vi "Lire_n_splits.vi"(8 "error in (no error)":errorcluster caption="entrée d'erreur (pas d'erreur)", 11 "Splitter en entrée":refnum<class "Splitter.lvclass">) -> (0 "error out":errorcluster caption="sortie d'erreur", 2 "n_splits":u8, 3 "Splitter en sortie":refnum<class "Splitter.lvclass">)   [LabVIEW 2020, in "Splitter.lvclass"]
uses:
  Splitter.lvclass
  Splitter.lvclass/Splitter.ctl
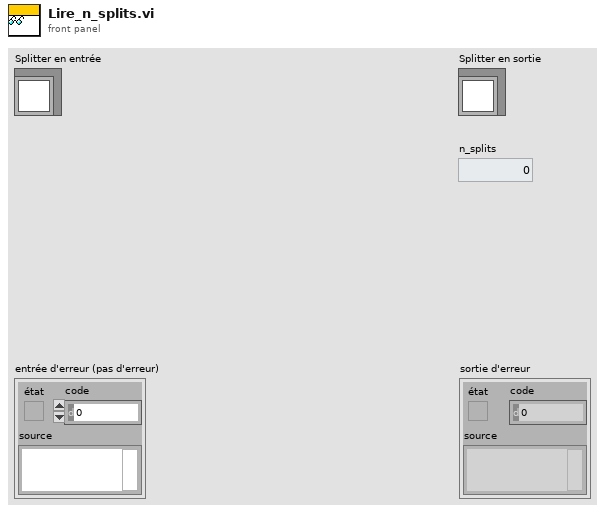
[diagram p1: front panel]
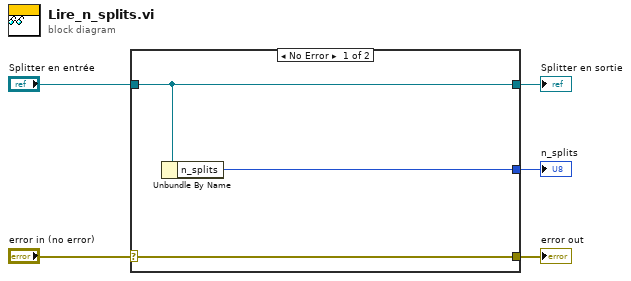
[diagram p0: block diagram]
diagram:
  n1 = case shown="No Error" "error in (no error)" {
    selector: "error in (no error)" -> [w8 w9]
    tunnel: [w8 w9] -> w4
    tunnel: [w7 w10] -> w2
    tunnel: "Splitter en entrée" -> [w7 w10]
    tunnel: [w6 _] -> w1
    frame No Error {
      n2 = Unbundle By Name(w7) -> ("n_splits"=w6:u8)
    }
    frame Error {
    }
  }
  "error out" <- w4
  "Splitter en sortie" <- w2
  "n_splits" <- w1
